vi "Log Close.vi"(10 "Log Handle In":T1, 11 "Error In":errorcluster) -> (3 "Error Out":errorcluster)   [LabVIEW 2021]
uses:
  Log Handle.ctl
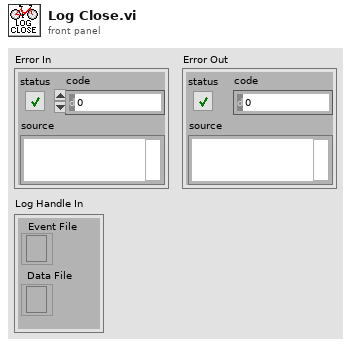
[diagram p1: front panel]
types:
  T1 = typedef "Log Handle.ctl" = cluster{"Data File":refnum<file>, "Event File":refnum<file>}
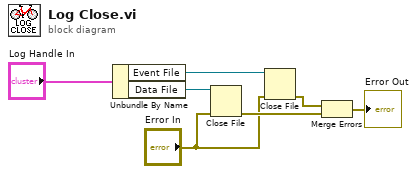
[diagram p0: block diagram]
diagram:
  n1 = Unbundle By Name("Log Handle In") -> ("Event File"=w5:refnum<file>, "Data File"=w6:refnum<file>)
  n2 = Close File(refnum=w6, error in="Error In") -> (error out=w4:errorcluster)  [unwired: 1 out]
  n3 = Close File(refnum=w5, error in="Error In") -> (error out=w3:errorcluster)  [unwired: 1 out]
  n4 = Merge Errors(w3, w4) -> (→"Error Out":errorcluster)
